vi "校准参数写入.vi"(8 "error in":errorcluster caption="错误输入", 9 "截距":dbl, 10 "斜率":dbl, 11 "Channel":u16=81 format="%.0x") -> (0 "error out":errorcluster caption="错误输出", 3 "Channel out":u16)   [LabVIEW 2020]
uses:
  <userlib>/PCANBasic/ctl/TPCANStatus.ctl
  <userlib>/PCANBasic/ctl/TPCANMsgFD.ctl
  <userlib>/PCANBasic/PCANBasic.lvlib
panel:
  out "TCANStatus 2":T1 items=["PCAN_ERROR_OK"=0, "PCAN_ERROR_XMTFULL"=1, "PCAN_ERROR_OVERRUN"=2, "PCAN_ERROR_BUSLIGHT"=4, "PCAN_ERROR_BUSHEAVY"=8, "PCAN_ERROR_BUSPASSIVE"=262144, "PCAN_ERROR_BUSOFF"=16, "PCAN_ERROR_QRCVEMPTY"=32, "PCAN_ERROR_QOVERRUN"=64, "PCAN_ERROR_QXMTFULL"=128, "PCAN_ERROR_REGTEST"=256, "PCAN_ERROR_NODRIVER"=512, "PCAN_ERROR_HWINUSE"=1024, "PCAN_ERROR_NETINUSE"=2048, "PCAN_ERROR_ILLHW"=5120, "PCAN_ERROR_ILLNET"=6144, "PCAN_ERROR_ILLCLIENT"=7168, "PCAN_ERROR_RESOURCE"=8192, "PCAN_ERROR_ILLPARAMTYPE"=16384, "PCAN_ERROR_ILLPARAMVAL"=32768, "PCAN_ERROR_UNKNOWN"=65536, "PCAN_ERROR_ILLDATA"=131072, "PCAN_ERROR_CAUTION"=33554432, "PCAN_ERROR_INITIALIZE"=67108864, "PCAN_ERROR_ILLOPERATION"=134217728]
  out "TCANStatus":T1 items=["PCAN_ERROR_OK"=0, "PCAN_ERROR_XMTFULL"=1, "PCAN_ERROR_OVERRUN"=2, "PCAN_ERROR_BUSLIGHT"=4, "PCAN_ERROR_BUSHEAVY"=8, "PCAN_ERROR_BUSPASSIVE"=262144, "PCAN_ERROR_BUSOFF"=16, "PCAN_ERROR_QRCVEMPTY"=32, "PCAN_ERROR_QOVERRUN"=64, "PCAN_ERROR_QXMTFULL"=128, "PCAN_ERROR_REGTEST"=256, "PCAN_ERROR_NODRIVER"=512, "PCAN_ERROR_HWINUSE"=1024, "PCAN_ERROR_NETINUSE"=2048, "PCAN_ERROR_ILLHW"=5120, "PCAN_ERROR_ILLNET"=6144, "PCAN_ERROR_ILLCLIENT"=7168, "PCAN_ERROR_RESOURCE"=8192, "PCAN_ERROR_ILLPARAMTYPE"=16384, "PCAN_ERROR_ILLPARAMVAL"=32768, "PCAN_ERROR_UNKNOWN"=65536, "PCAN_ERROR_ILLDATA"=131072, "PCAN_ERROR_CAUTION"=33554432, "PCAN_ERROR_INITIALIZE"=67108864, "PCAN_ERROR_ILLOPERATION"=134217728]
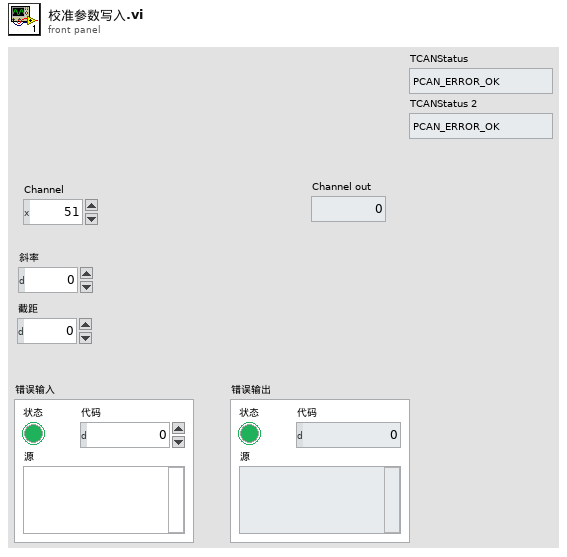
[diagram p1: front panel]
types:
  T1 = typedef "PCANBasic.lvlib/TPCANStatus.ctl" = u32
  T2 = typedef "PCANBasic.lvlib/TPCANMsgFD.ctl" = cluster{"ID":u32, "MSGTYPE":u8, "DLC":u8, "DATA":cluster{"[0]":u8, "[1]":u8, "[2]":u8, "[3]":u8, "[4]":u8, "[5]":u8, "[6]":u8, "[7]":u8, "[8]":u8, "[9]":u8, "[10]":u8, "[11]":u8, "[12]":u8, "[13]":u8, "[14]":u8, "[15]":u8, "[16]":u8, "[17]":u8, "[18]":u8, "[19]":u8, "[20]":u8, "[21]":u8, "[22]":u8, "[23]":u8, "[24]":u8, "[25]":u8, "[26]":u8, "[27]":u8, "[28]":u8, "[29]":u8, "[30]":u8, "[31]":u8, "[32]":u8, "[33]":u8, "[34]":u8, "[35]":u8, "[36]":u8, "[37]":u8, "[38]":u8, "[39]":u8, "[40]":u8, "[41]":u8, "[42]":u8, "[43]":u8, "[44]":u8, "[45]":u8, "[46]":u8, "[47]":u8, "[48]":u8, "[49]":u8, "[50]":u8, "[51]":u8, "[52]":u8, "[53]":u8, "[54]":u8, "[55]":u8, "[56]":u8, "[57]":u8, "[58]":u8, "[59]":u8, "[60]":u8, "[61]":u8, "[62]":u8, "[63]":u8}}
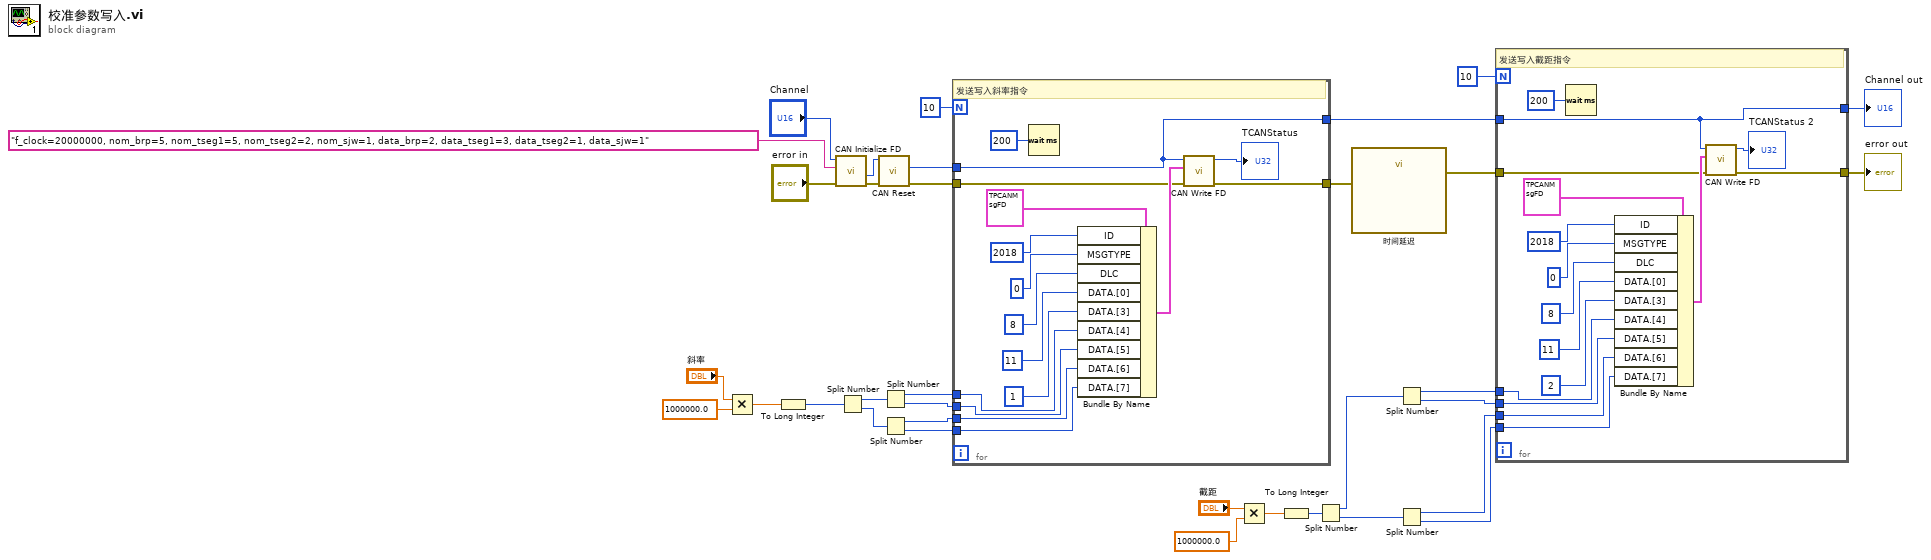
[diagram p0: block diagram]
diagram:
  n1 = Multiply(x="斜率", y=1000000.0) -> (x*y=w9:dbl)
  n2 = To Long Integer(number=w9) -> (32bit integer=w8:i32)
  n3 = call <userlib>:"CAN Initialize FD.vi"("error in"="error in", "BitrateFD"="f_clock=20000000, nom_brp=5, nom_tseg1=5, nom_tseg2=2, nom_sjw=1, data_brp=2, data_tseg1=3, data_tseg2=1, data_sjw=1", "Channel"="Channel") -> ("error out"=w12:errorcluster, "Channel out"=w31:u16)  [unwired: 5 in, 2 out]
  n4 = Split Number(x=w8) -> (hi(x)=w29:u16, lo(x)=w28:u16)
  n5 = call <userlib>:"CAN Reset.vi"("错误输入（无错误）"=w12, "Channel in"=w31) -> ("错误输出"=w11:errorcluster, "Channel out"=w30:u16)  [unwired: 7 in, 1 out]
  n6 = Split Number(x=w29) -> (hi(x)=w27:u8, lo(x)=w26:u8)
  n7 = Split Number(x=w28) -> (hi(x)=w25:u8, lo(x)=w24:u8)
  n8 = for {
    N: 10 -> [_]
    tunnel: w30 -> [w48]
    tunnel: [w48] -> w17
    tunnel: w27 -> [w43]
    tunnel: w26 -> [w42]
    tunnel: w25 -> [w41]
    tunnel: w24 -> [w40]
    tunnel: [w37] -> w1
    tunnel: w11 -> [w36]
    # "发送写入斜率指令"
    n9 = Wait (ms)(milliseconds to wait=u32 200 ("等待时间（毫秒）")) -> ()  [unwired: 1 out]
    n10 = Bundle By Name(cluster=T2 {"ID"=0, "MSGTYPE"=0, "DLC"=0, "DATA"={"[0]"=0, "[1]"=0, "[2]"=0, "[3]"=0, "[4]"=0, "[5]"=0, "[6]"=0, "[7]"=0, "[8]"=0, "[9]"=0, "[10]"=0, "[11]"=0, "[12]"=0, "[13]"=0, "[14]"=0, "[15]"=0, "[16]"=0, "[17]"=0, "[18]"=0, "[19]"=0, "[20]"=0, "[21]"=0, "[22]"=0, "[23]"=0, "[24]"=0, "[25]"=0, "[26]"=0, "[27]"=0, "[28]"=0, "[29]"=0, "[30]"=0, "[31]"=0, "[32]"=0, "[33]"=0, "[34]"=0, "[35]"=0, "[36]"=0, "[37]"=0, "[38]"=0, "[39]"=0, "[40]"=0, "[41]"=0, "[42]"=0, "[43]"=0, "[44]"=0, "[45]"=0, "[46]"=0, "[47]"=0, "[48]"=0, "[49]"=0, "[50]"=0, "[51]"=0, "[52]"=0, "[53]"=0, "[54]"=0, "[55]"=0, "[56]"=0, "[57]"=0, "[58]"=0, "[59]"=0, "[60]"=0, "[61]"=0, "[62]"=0, "[63]"=0}} ("MessageBuffer in"), "ID"=u32 2018, "MSGTYPE"=u8 0, "DLC"=u8 8 ("ID"), "DATA.[0]"=u8 11 ("ID"), "DATA.[3]"=u8 1 ("DATA[3]"), "DATA.[4]"=w43, "DATA.[5]"=w42, "DATA.[6]"=w41, "DATA.[7]"=w40) -> (w38:T2)
    n11 = call <userlib>:"CAN Write FD.vi"("错误输入（无错误）"=w36, "MessageBuffer in"=w38, "Channel"=w48) -> ("错误输出"=w37:errorcluster, "TCANStatus"=→"TCANStatus":T1)  [unwired: 5 in, 2 out]
  }
  n12 = Multiply(x="截距", y=1000000.0) -> (x*y=w5:dbl)
  n13 = To Long Integer(number=w5) -> (32bit integer=w3:i32)
  n14 = Split Number(x=w3) -> (hi(x)=w22:u16, lo(x)=w23:u16)
  n15 = call "时间延迟"("error in (no error)"=w1) -> ("error out"=w2:errorcluster)  [unwired: 10 in]
  n16 = Split Number(x=w22) -> (hi(x)=w21:u8, lo(x)=w20:u8)
  n17 = Split Number(x=w23) -> (hi(x)=w19:u8, lo(x)=w18:u8)
  n18 = for {
    N: 10 -> [_]
    tunnel: w17 -> [w64]
    tunnel: [w64] -> w15
    tunnel: w21 -> [w58]
    tunnel: w20 -> [w57]
    tunnel: w19 -> [w56]
    tunnel: w18 -> [w55]
    tunnel: [w53] -> w14
    tunnel: w2 -> [w52]
    # "发送写入截距指令"
    n19 = Wait (ms)(milliseconds to wait=u32 200 ("等待时间（毫秒）")) -> ()  [unwired: 1 out]
    n20 = Bundle By Name(cluster=T2 {"ID"=0, "MSGTYPE"=0, "DLC"=0, "DATA"={"[0]"=0, "[1]"=0, "[2]"=0, "[3]"=0, "[4]"=0, "[5]"=0, "[6]"=0, "[7]"=0, "[8]"=0, "[9]"=0, "[10]"=0, "[11]"=0, "[12]"=0, "[13]"=0, "[14]"=0, "[15]"=0, "[16]"=0, "[17]"=0, "[18]"=0, "[19]"=0, "[20]"=0, "[21]"=0, "[22]"=0, "[23]"=0, "[24]"=0, "[25]"=0, "[26]"=0, "[27]"=0, "[28]"=0, "[29]"=0, "[30]"=0, "[31]"=0, "[32]"=0, "[33]"=0, "[34]"=0, "[35]"=0, "[36]"=0, "[37]"=0, "[38]"=0, "[39]"=0, "[40]"=0, "[41]"=0, "[42]"=0, "[43]"=0, "[44]"=0, "[45]"=0, "[46]"=0, "[47]"=0, "[48]"=0, "[49]"=0, "[50]"=0, "[51]"=0, "[52]"=0, "[53]"=0, "[54]"=0, "[55]"=0, "[56]"=0, "[57]"=0, "[58]"=0, "[59]"=0, "[60]"=0, "[61]"=0, "[62]"=0, "[63]"=0}} ("MessageBuffer in"), "ID"=u32 2018, "MSGTYPE"=u8 0, "DLC"=u8 8 ("ID"), "DATA.[0]"=u8 11 ("ID"), "DATA.[3]"=u8 2 ("DATA[3]"), "DATA.[4]"=w58, "DATA.[5]"=w57, "DATA.[6]"=w56, "DATA.[7]"=w55) -> (w59:T2)
    n21 = call <userlib>:"CAN Write FD.vi"("错误输入（无错误）"=w52, "MessageBuffer in"=w59, "Channel"=w64) -> ("错误输出"=w53:errorcluster, "TCANStatus"=→"TCANStatus 2":T1)  [unwired: 5 in, 2 out]
  }
  "Channel out" <- w15
  "error out" <- w14
